vi "siMPx Func Encode coordinates (microsteps) before sending.vi"(1 "Z microsteps":i32, 2 "Y microsteps":i32, 3 "X microsteps":i32) -> (0 "Coordinates string ready to send":string)   [LabVIEW 2015, in "XYZStage.lvlib"]
doc: "This SubVI extracts two bytes from specific points in a string, swaps the bytes, and then combines them into a single 16-bit word unsigned integer.\nInputs: String, 1st offset, 2nd offset\nOutputs: 16-bit unsigned integer."
uses:
  XYZStage.lvlib
panel:
  # "Function to reverse the bytes of MP-285 or MPC-200 X, Y, & Z coordinates (in microsteps), convert each to strings, then concatenate them into a single string ready for sending to the conroller."
  # "INPUT"
  # "OUTPUT"
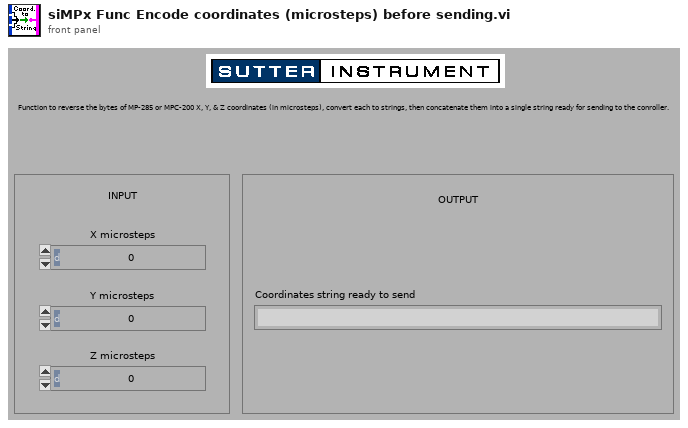
[diagram p1: front panel]
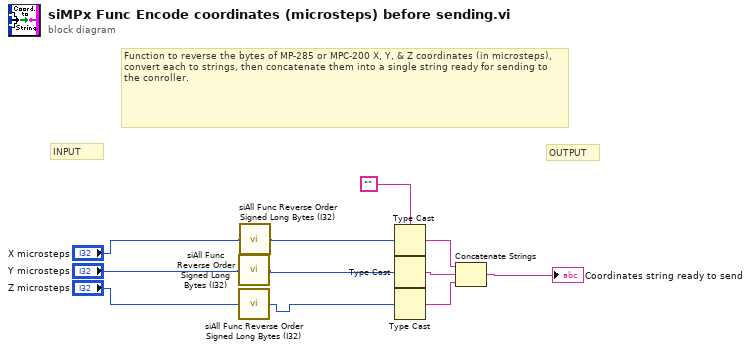
[diagram p0: block diagram]
diagram:
  w8 = "" ("String type")
  # "OUTPUT"
  # "INPUT"
  # "Function to reverse the bytes of MP-285 or MPC-200 X, Y, & Z coordinates (in microsteps), convert each to strings, then concatenate them into a single string ready for sending to the conroller."
  n1 = call "siAll Func Reverse Order Signed Long Bytes (I32).vi"("Input I32 to convert"="Y microsteps") -> ("Output I32 with byte order reversed"=w4:i32)
  n2 = call "siAll Func Reverse Order Signed Long Bytes (I32).vi"("Input I32 to convert"="Z microsteps") -> ("Output I32 with byte order reversed"=w2:i32)
  n3 = call "siAll Func Reverse Order Signed Long Bytes (I32).vi"("Input I32 to convert"="X microsteps") -> ("Output I32 with byte order reversed"=w6:i32)
  n4 = Type Cast ("Convert to string")(type=w8, x=w6) -> (*(type *) &x=w11:string)
  n5 = Type Cast(type=w8, x=w4) -> (*(type *) &x=w10:string)
  n6 = Type Cast(type=w8, x=w2) -> (*(type *) &x=w9:string)
  n7 = Concatenate Strings ("Concatenate strings into one command sequence")(w11, w10, w9) -> (→"Coordinates string ready to send":string)
